vi "Start Sync.vi"(8 "error in (no error)":errorcluster, 10 "current time":timestamp, 11 "gRPC Server in":refnum<class "HVC8.lvclass">) -> (0 "error out":errorcluster, 3 "gRPC Server out":refnum<class "HVC8.lvclass">)   [LabVIEW 2019, in "HVC8.lvlib" / "HVC8.lvclass"]
uses:
  HVC8.lvclass
  DIOSessions.ctl
  DISession.ctl
  DOSession.ctl
  HVC8.lvclass/HVC8.ctl
  RPC Messages/measurementservice_QueryResponse/measurementservice_QueryResponse_Data.ctl
  RPC Messages/measurementservice_DIOpenSessionResponse/measurementservice_DIOpenSessionResponse_Data.ctl
  RPC Messages/measurementservice_ErrorOut/measurementservice_ErrorOut_Data.ctl
  RPC Messages/measurementservice_ReadDIResponse/measurementservice_ReadDIResponse_Data.ctl
  RPC Messages/measurementservice_DICloseSessionResponse/measurementservice_DICloseSessionResponse_Data.ctl
  RPC Messages/measurementservice_DOOpenSessionResponse/measurementservice_DOOpenSessionResponse_Data.ctl
  RPC Messages/measurementservice_DOCloseSessionResponse/measurementservice_DOCloseSessionResponse_Data.ctl
  RPC Messages/measurementservice_WriteDOResponse/measurementservice_WriteDOResponse_Data.ctl
  <vilib>/DAQmx/read.llb/DAQmx Read (Digital 1D Bool 1Chan 1Samp).vi
  <vilib>/DAQmx/write.llb/DAQmx Write (Digital 1D Bool 1Chan 1Samp).vi
  <vilib>/DAQmx/create/channels.llb/DAQmx Create Channel (DI-Digital Input).vi
  <vilib>/DAQmx/miscellaneous.llb/DAQmx Fill In Error Info.vi
  <vilib>/DAQmx/create/channels.llb/DAQmx Create Channel (DO-Digital Output).vi
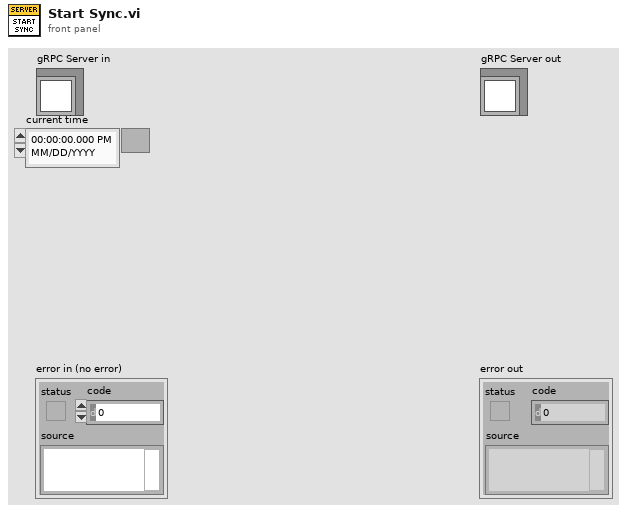
[diagram p1: front panel]
types:
  T1 = typedef "HVC8.lvlib/HVC8.lvclass/DIOSessions.ctl" = cluster{"Array of DI Sessions":T2[], "Array of DO Sessions":T3[]}
  T2 = typedef "HVC8.lvlib/HVC8.lvclass/DISession.ctl" = cluster{"DI Task":refnum<k21>, "DISessionName":string}
  T3 = typedef "HVC8.lvlib/HVC8.lvclass/DOSession.ctl" = cluster{"DOTask":refnum<k21>, "DOSessionName":string}
  T4 = typedef "HVC8.lvlib/HVC8.lvclass/measurementservice_QueryResponse_Data.ctl" = cluster{"message":string, "status":i32}
  T5 = typedef "HVC8.lvlib/HVC8.lvclass/measurementservice_ErrorOut_Data.ctl" = cluster{"errCode":i32, "errMessage":string}
  T6 = typedef "HVC8.lvlib/HVC8.lvclass/measurementservice_DIOpenSessionResponse_Data.ctl" = cluster{"DISessionName":string, "error":T5}
  T7 = typedef "HVC8.lvlib/HVC8.lvclass/measurementservice_ReadDIResponse_Data.ctl" = cluster{"DIOSessionName":string, "DIData":bool[], "error":T5}
  T8 = typedef "HVC8.lvlib/HVC8.lvclass/measurementservice_DICloseSessionResponse_Data.ctl" = cluster{"error":T5}
  T9 = typedef "HVC8.lvlib/HVC8.lvclass/measurementservice_DOOpenSessionResponse_Data.ctl" = cluster{"DOSessionName":string, "error":T5}
  T10 = typedef "HVC8.lvlib/HVC8.lvclass/measurementservice_DOCloseSessionResponse_Data.ctl" = cluster{"error":T5}
  T11 = typedef "HVC8.lvlib/HVC8.lvclass/measurementservice_WriteDOResponse_Data.ctl" = cluster{"DIOSessionName":string, "error":T5}
  T12 = typedef "HVC8.lvlib/HVC8.lvclass/Server gRPC UEs.ctl" = cluster{"Invoke gRPC UE":refnum<user-event>, "Query gRPC UE":refnum<user-event>, "Register gRPC UE":refnum<user-event>, "OpenDISession gRPC UE":refnum<user-event>, "OpenDOSession gRPC UE":refnum<user-event>, "ReadDI gRPC UE":refnum<user-event>, "WriteDO gRPC UE":refnum<user-event>, "CloseDISession gRPC UE":refnum<user-event>, "CloseDOSession gRPC UE":refnum<user-event>}
  T13 = typedef "HVC8.lvlib/gprc-lvsupport.lvlib/grpcId.ctl" = u64
  T14 = typedef "HVC8.lvlib/HVC8.lvclass/measurementservice_QueryRequest_Data.ctl" = cluster{"query":string}
  T15 = typedef "HVC8.lvlib/HVC8.lvclass/measurementservice_DIOpenSessionRequest_Data.ctl" = cluster{"DISessionName":string, "DIlines":string}
  T16 = typedef "HVC8.lvlib/HVC8.lvclass/measurementservice_ReadDIRequest_Data.ctl" = cluster{"DIOSessionName":string}
  T17 = typedef "HVC8.lvlib/HVC8.lvclass/measurementservice_DICloseSessionRequest_Data.ctl" = cluster{"DISessionName":string}
  T18 = typedef "HVC8.lvlib/HVC8.lvclass/measurementservice_DOOpenSessionRequest_Data.ctl" = cluster{"DOSessionName":string, "DOlines":string}
  T19 = typedef "HVC8.lvlib/HVC8.lvclass/measurementservice_DOCloseSessionRequest_Data.ctl" = cluster{"DOSessionName":string}
  T20 = typedef "HVC8.lvlib/HVC8.lvclass/measurementservice_WriteDORequest_Data.ctl" = cluster{"DIOSessionName":string, "DOData":bool[]}
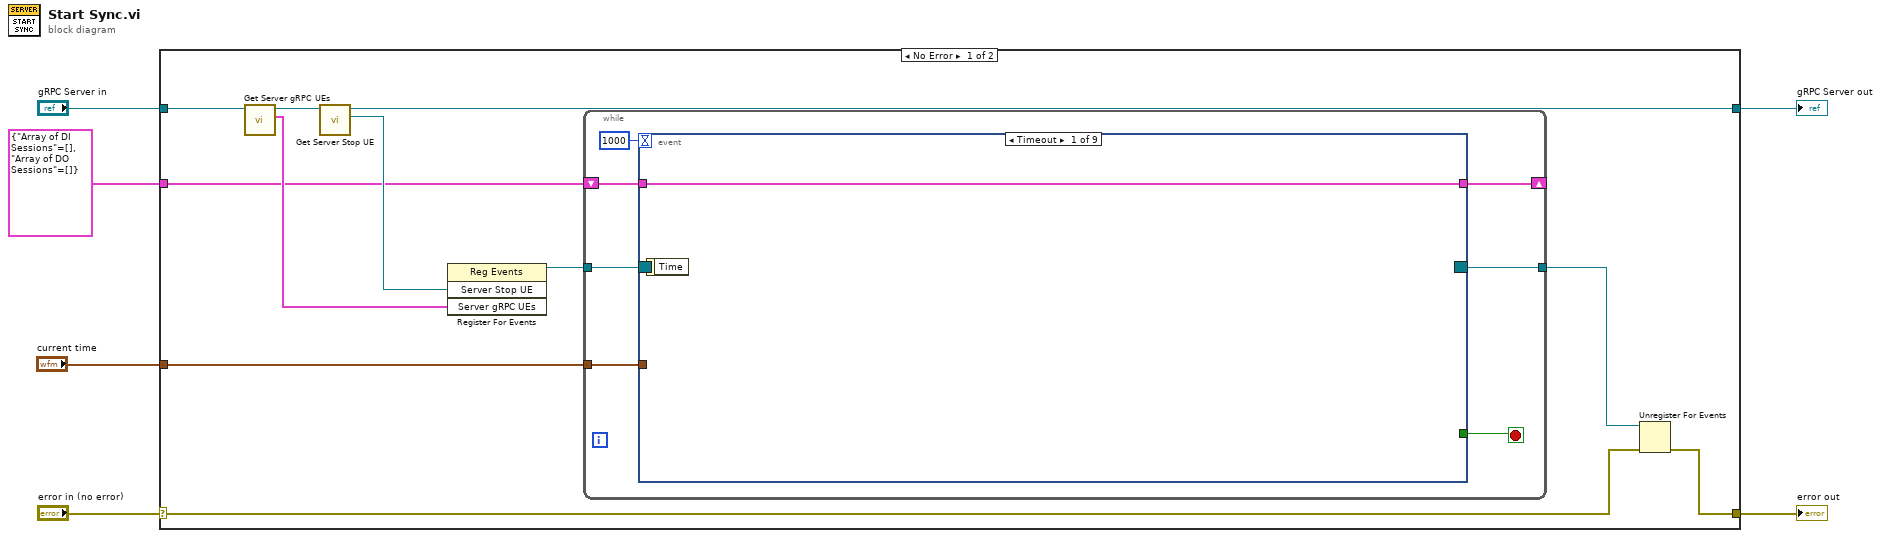
[diagram p0: block diagram]
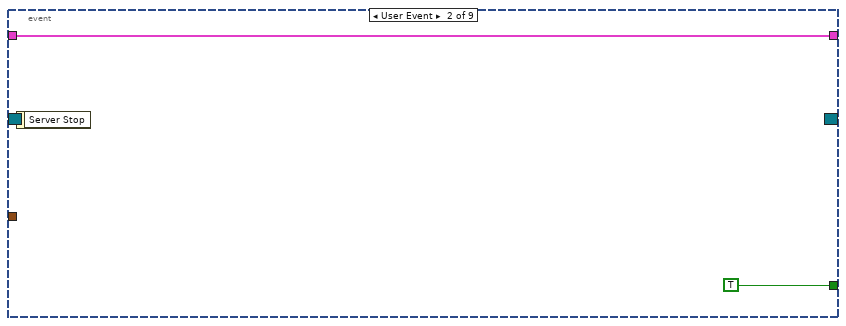
[diagram p2: hidden frame]
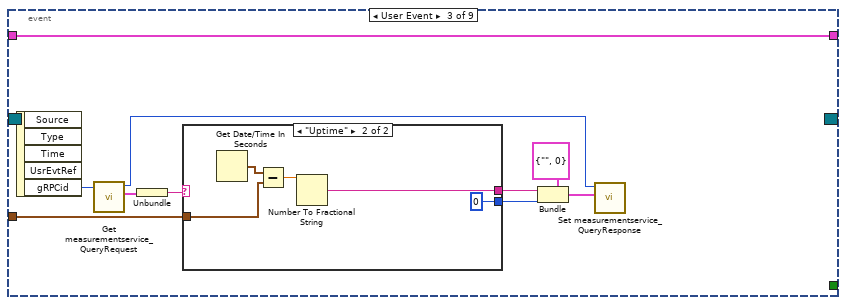
[diagram p3: hidden frame]
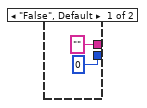
[diagram p4: hidden frame]
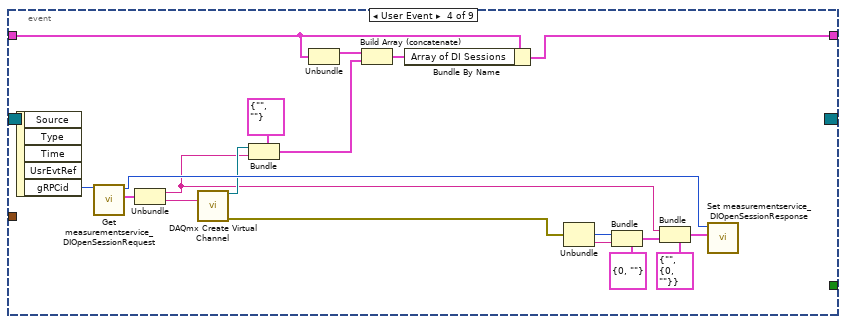
[diagram p5: hidden frame]
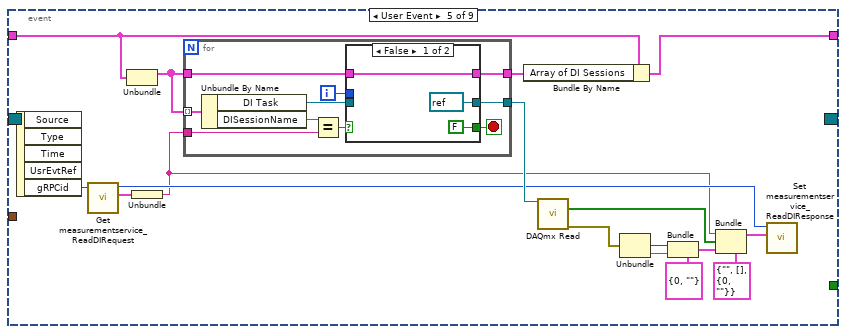
[diagram p6: hidden frame]
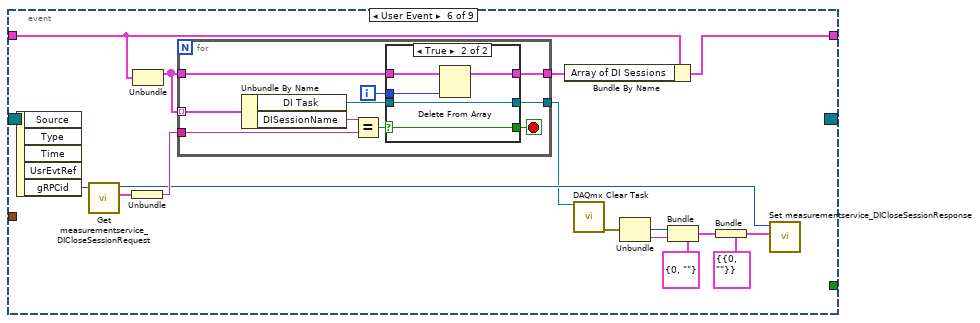
[diagram p8: hidden frame]
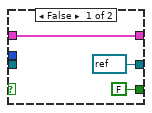
[diagram p9: hidden frame]
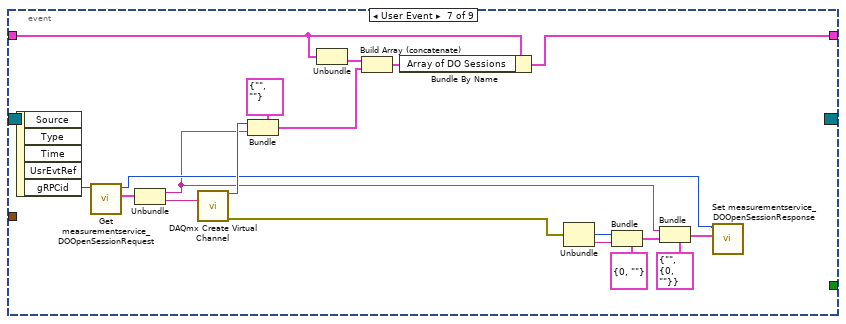
[diagram p10: hidden frame]
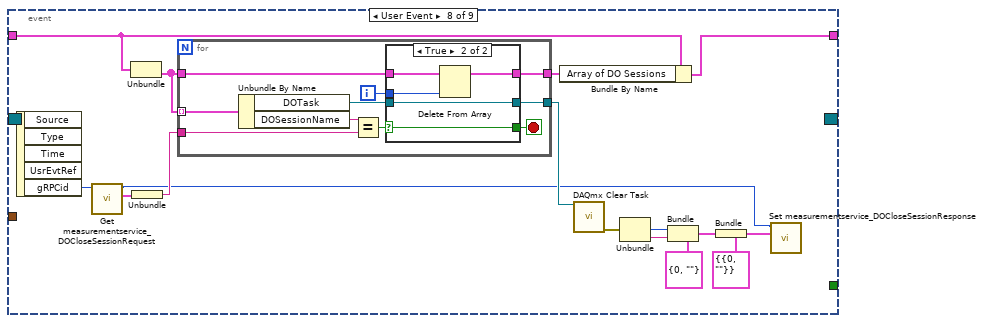
[diagram p11: hidden frame]
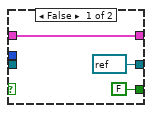
[diagram p12: hidden frame]
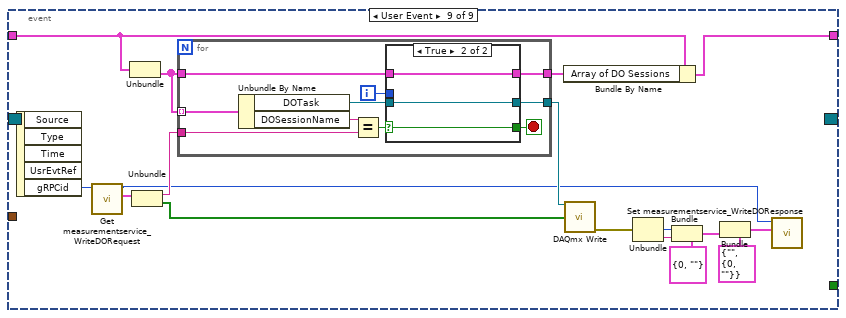
[diagram p13: hidden frame]
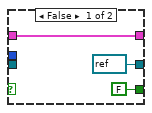
[diagram p14: hidden frame]
diagram:
  n1 = case shown="No Error" "error in (no error)" {
    selector: "error in (no error)" -> [w10 w218]
    tunnel: [w9 w218] -> w5
    tunnel: [w13 w217] -> w3
    tunnel: "gRPC Server in" -> [w17 w217]
    tunnel: "current time" -> [w8 _]
    tunnel: T1 {"Array of DI Sessions"=[], "Array of DO Sessions"=[]} -> [w7 _]
    frame No Error {
      n2 = call "Get Server gRPC UEs.vi"("OOP Server in"=w17) -> ("Server gRPC UEs"=w14:T12, "OOP Server out"=w16:refnum<class "HVC8.lvclass">)  [unwired: 9 in]
      n3 = call "Get Server Stop UE.vi"("OOP Server in"=w16) -> ("Server Stop UE"=w15:refnum<user-event>, "OOP Server out"=w13:refnum<class "HVC8.lvclass">)  [unwired: 9 in]
      n4 = register-events(w15, w14) -> (reference out=w12:refnum<event-registration>)  [unwired: 2 in, 1 out]
      n5 = while {
        tunnel: w12 -> [w24]
        tunnel: [w22] -> w11
        tunnel: w8 -> [w20]
        shift-right: [w18] -> _
        shift-left: w7 -> [w19]
        stop <- w23 stop-if-true
        n6 = event "RPC Methods Event Structure" shown="[0] Timeout" {
          selector: w24 -> [_ _ _ _ _ _ _ _ _]
          dyn-events: [_ _ _ _ _ _ _ _ _] -> w22
          timeout: 1000 -> [_ _ _ _ _ _ _ _ _]
          tunnel: [_ TRUE _ _ _ _ _ _ _] -> w23
          tunnel: w20 -> [_ _ w31 _ _ _ _ _ _]
          tunnel: w19 -> [w25 w26 w28 w47 w66 w99 w131 w152 w185]
          tunnel: [w25 w26 w28 w46 w65 w98 w133 w151 w184] -> w18
          event Timeout {
            n7 = event-data() -> ()  [unwired: 1 in, 1 out]
          }
          event User Event {
            n8 = event-data() -> ()  [unwired: 1 in, 1 out]
          }
          event User Event {
            n9 = event-data() -> ("gRPCid"=w35:T13)  [unwired: 1 in, 4 out]
            n10 = call "Get measurementservice_QueryRequest.vi"("gRPCid"=w35) -> ("Message Data"=w34:T14, "gRPCid out"=w33:T13)  [unwired: 8 in, 1 out]
            n11 = Unbundle(w34) -> ("query"=w32:string)
            n12 = case shown="\"Uptime\"" w32 {
              tunnel: w31 -> [_ w43]
              tunnel: ["" w41] -> w30
              tunnel: [0 ("status") 0 ("status")] -> w29
              frame "False", Default {
              }
              frame "Uptime" {
                n13 = Get Date/Time In Seconds() -> (seconds since 1Jan1904=w44:timestamp)
                n14 = Subtract(x=w44, y=w43) -> (x-y=w42:dbl)
                n15 = Number To Fractional String(number=w42) -> (F-format string=w41:string)  [unwired: 3 in]
              }
            }
            n16 = Bundle(cluster=T4 {"message"="", "status"=0} ("measurementservice_QueryResponse_Data"), "message"=w30, "status"=w29) -> (w36:T4)
            n17 = call "Set measurementservice_QueryResponse.vi"("Message Data"=w36, "gRPCid"=w33) -> ()  [unwired: 9 in, 1 out]
          }
          event User Event {
            n18 = event-data() -> ("gRPCid"=w59:T13)  [unwired: 1 in, 4 out]
            n19 = call "Get measurementservice_DIOpenSessionRequest.vi"("gRPCid"=w59) -> ("Message Data"=w58:T15, "gRPCid out"=w57:T13)  [unwired: 8 in, 1 out]
            n20 = Unbundle(w58) -> ("DISessionName"=w48:string, "DIlines"=w56:string)
            n21 = call-poly <vilib>:"DAQmx Create Virtual Channel.vi"("lines"=w56) -> ("task out"=w49:refnum<k21>, "error out"=w55:errorcluster)  [unwired: 13 in]
            n22 = Bundle(cluster=T2 {"DI Task"="", "DISessionName"=""}, "DI Task"=w49, "DISessionName"=w48) -> (w50:T2)
            n23 = Unbundle(w47) -> ("Array of DI Sessions"=w51:T2[])  [unwired: 1 out]
            n24 = Build Array (concatenate)(w51, w50) -> (w45:T2[])
            n25 = Bundle By Name(cluster=w47, "Array of DI Sessions"=w45) -> (w46:T1)
            n26 = Unbundle(w55) -> ("code"=w54:i32, "source"=w53:string)  [unwired: 1 out]
            n27 = Bundle(cluster=T5 {"errCode"=0, "errMessage"=""} ("error"), "errCode"=w54, "errMessage"=w53) -> (w60:T5)
            n28 = Bundle(cluster=T6 {"DISessionName"="", "error"={"errCode"=0, "errMessage"=""}} ("measurementservice_DIOpenSessionResponse_Data"), "DISessionName"=w48, "error"=w60) -> (w62:T6)
            n29 = call "Set measurementservice_DIOpenSessionResponse.vi"("Message Data"=w62, "gRPCid"=w57) -> ()  [unwired: 9 in, 1 out]
          }
          event User Event {
            n30 = event-data() -> ("gRPCid"=w75:T13)  [unwired: 1 in, 4 out]
            n31 = call "Get measurementservice_ReadDIRequest.vi"("gRPCid"=w75) -> ("Message Data"=w74:T16, "gRPCid out"=w73:T13)  [unwired: 8 in, 1 out]
            n32 = Unbundle(w66) -> ("Array of DI Sessions"=w78:T2[])  [unwired: 1 out]
            n33 = Unbundle(w74) -> ("DIOSessionName"=w67:string)
            n34 = for {
              tunnel: w78 -> [w85] mode=indexing
              tunnel: w67 -> [w90]
              tunnel: [w86] -> w77
              tunnel: w78 -> [w84]
              tunnel: [w83] -> w64
              i -> [w81]
              stop <- w88 stop-if-true
              n35 = Unbundle By Name(w85) -> ("DI Task"=w87:refnum<k21>, "DISessionName"=w82:string)
              n36 = Equal?(x=w82, y=w90) -> (x = y?=w89:bool)
              n37 = case shown="False" w89 {
                selector: w89 -> [_ w96]
                tunnel: [FALSE w96] -> w88
                tunnel: w87 -> [_ w94]
                tunnel: [refnum<k21> refnum ("DI Task") w94] -> w86
                tunnel: w84 -> [w91 w95]
                tunnel: [w91 w95] -> w83
                tunnel: w81 -> [_ _]
                frame False {
                }
                frame True {
                }
              }
            }
            n38 = Bundle By Name(cluster=w66, "Array of DI Sessions"=w64) -> (w65:T1)
            n39 = call-poly <vilib>:"DAQmx Read.vi"("task/channels in"=w77) -> ("data"=w68:bool[], "error out"=w76:errorcluster)  [unwired: 12 in, 1 out]
            n40 = Unbundle(w76) -> ("code"=w80:i32, "source"=w79:string)  [unwired: 1 out]
            n41 = Bundle(cluster=T5 {"errCode"=0, "errMessage"=""} ("error"), "errCode"=w80, "errMessage"=w79) -> (w69:T5)
            n42 = Bundle(cluster=T7 {"DIOSessionName"="", "DIData"=[], "error"={"errCode"=0, "errMessage"=""}} ("measurementservice_ReadDIResponse_Data"), "DIOSessionName"=w67, "DIData"=w68, "error"=w69) -> (w72:T7)
            n43 = call "Set measurementservice_ReadDIResponse.vi"("Message Data"=w72, "gRPCid"=w73) -> ()  [unwired: 9 in, 1 out]
          }
          event User Event {
            n44 = event-data() -> ("gRPCid"=w109:T13)  [unwired: 1 in, 4 out]
            n45 = call "Get measurementservice_DICloseSessionRequest.vi"("gRPCid"=w109) -> ("Message Data"=w108:T17, "gRPCid out"=w106:T13)  [unwired: 8 in, 1 out]
            n46 = Unbundle(w108) -> ("DISessionName"=w107:string)
            n47 = Unbundle(w99) -> ("Array of DI Sessions"=w100:T2[])  [unwired: 1 out]
            n48 = for {
              tunnel: w100 -> [w117] mode=indexing
              tunnel: w107 -> [w122]
              tunnel: [w118] -> w101
              tunnel: w100 -> [w116]
              tunnel: [w115] -> w97
              i -> [w113]
              stop <- w120 stop-if-true
              n49 = Unbundle By Name(w117) -> ("DI Task"=w119:refnum<k21>, "DISessionName"=w114:string)
              n50 = Equal?(x=w114, y=w122) -> (x = y?=w121:bool)
              n51 = case shown="True" w121 {
                selector: w121 -> [_ w130]
                tunnel: [FALSE w130] -> w120
                tunnel: w119 -> [_ w128]
                tunnel: [refnum<k21> refnum ("DI Task") w128] -> w118
                tunnel: w116 -> [w123 w129]
                tunnel: [w123 w126] -> w115
                tunnel: w113 -> [_ w127]
                frame False {
                }
                frame True {
                  n52 = Delete From Array(array=w129, index=w127) -> (array with subset deleted=w126:T2[])  [unwired: 1 in, 1 out]
                }
              }
            }
            n53 = Bundle By Name(cluster=w99, "Array of DI Sessions"=w97) -> (w98:T1)
            n54 = call <vilib>:"DAQmx Clear Task.vi"("task in"=w101) -> ("error out"=w110:errorcluster)  [unwired: 14 in]
            n55 = Unbundle(w110) -> ("code"=w112:i32, "source"=w111:string)  [unwired: 1 out]
            n56 = Bundle(cluster=T5 {"errCode"=0, "errMessage"=""} ("error"), "errCode"=w112, "errMessage"=w111) -> (w102:T5)
            n57 = Bundle(cluster=T8 {"error"={"errCode"=0, "errMessage"=""}} ("measurementservice_DICloseSessionResponse_Data"), "error"=w102) -> (w105:T8)
            n58 = call "Set measurementservice_DICloseSessionResponse.vi"("Message Data"=w105, "gRPCid"=w106) -> ()  [unwired: 9 in, 1 out]
          }
          event User Event {
            n59 = event-data() -> ("gRPCid"=w144:T13)  [unwired: 1 in, 4 out]
            n60 = call "Get measurementservice_DOOpenSessionRequest.vi"("gRPCid"=w144) -> ("Message Data"=w143:T18, "gRPCid out"=w139:T13)  [unwired: 8 in, 1 out]
            n61 = Unbundle(w143) -> ("DOSessionName"=w134:string, "DOlines"=w149:string)
            n62 = call-poly <vilib>:"DAQmx Create Virtual Channel.vi"("lines"=w149) -> ("task out"=w145:refnum<k21>, "error out"=w148:errorcluster)  [unwired: 13 in]
            n63 = Bundle(cluster=T3 {"DOTask"="", "DOSessionName"=""} ("output cluster"), "DOTask"=w145, "DOSessionName"=w134) -> (w140:T3)
            n64 = Unbundle(w131) -> ("Array of DO Sessions"=w142:T3[])  [unwired: 1 out]
            n65 = Build Array (concatenate)(w142, w140) -> (w132:T3[])
            n66 = Bundle By Name(cluster=w131, "Array of DO Sessions"=w132) -> (w133:T1)
            n67 = Unbundle(w148) -> ("code"=w147:i32, "source"=w146:string)  [unwired: 1 out]
            n68 = Bundle(cluster=T5 {"errCode"=0, "errMessage"=""} ("error"), "errCode"=w147, "errMessage"=w146) -> (w135:T5)
            n69 = Bundle(cluster=T9 {"DOSessionName"="", "error"={"errCode"=0, "errMessage"=""}} ("measurementservice_DOOpenSessionResponse_Data"), "DOSessionName"=w134, "error"=w135) -> (w138:T9)
            n70 = call "Set measurementservice_DOOpenSessionResponse.vi"("Message Data"=w138, "gRPCid"=w139) -> ()  [unwired: 9 in, 1 out]
          }
          event User Event {
            n71 = event-data() -> ("gRPCid"=w160:T13)  [unwired: 1 in, 4 out]
            n72 = call "Get measurementservice_DOCloseSessionRequest.vi"("gRPCid"=w160) -> ("Message Data"=w159:T19, "gRPCid out"=w158:T13)  [unwired: 8 in, 1 out]
            n73 = Unbundle(w152) -> ("Array of DO Sessions"=w153:T3[])  [unwired: 1 out]
            n74 = Unbundle(w159) -> ("DOSessionName"=w162:string)
            n75 = for {
              tunnel: w153 -> [w170] mode=indexing
              tunnel: w162 -> [w175]
              tunnel: [w171] -> w161
              tunnel: w153 -> [w169]
              tunnel: [w168] -> w150
              i -> [w166]
              stop <- w173 stop-if-true
              n76 = Unbundle By Name(w170) -> ("DOTask"=w172:refnum<k21>, "DOSessionName"=w167:string)
              n77 = Equal?(x=w167, y=w175) -> (x = y?=w174:bool)
              n78 = case shown="True" w174 {
                selector: w174 -> [_ w183]
                tunnel: [FALSE w183] -> w173
                tunnel: w172 -> [_ w181]
                tunnel: [refnum<k21> refnum ("DI Task") w181] -> w171
                tunnel: w169 -> [w176 w182]
                tunnel: [w176 w179] -> w168
                tunnel: w166 -> [_ w180]
                frame False {
                }
                frame True {
                  n79 = Delete From Array(array=w182, index=w180) -> (array with subset deleted=w179:T3[])  [unwired: 1 in, 1 out]
                }
              }
            }
            n80 = Bundle By Name(cluster=w152, "Array of DO Sessions"=w150) -> (w151:T1)
            n81 = call <vilib>:"DAQmx Clear Task.vi"("task in"=w161) -> ("error out"=w163:errorcluster)  [unwired: 14 in]
            n82 = Unbundle(w163) -> ("code"=w165:i32, "source"=w164:string)  [unwired: 1 out]
            n83 = Bundle(cluster=T5 {"errCode"=0, "errMessage"=""} ("error"), "errCode"=w165, "errMessage"=w164) -> (w154:T5)
            n84 = Bundle(cluster=T10 {"error"={"errCode"=0, "errMessage"=""}} ("measurementservice_DOCloseSessionResponse_Data"), "error"=w154) -> (w156:T10)
            n85 = call "Set measurementservice_DOCloseSessionResponse.vi"("Message Data"=w156, "gRPCid"=w158) -> ()  [unwired: 9 in, 1 out]
          }
          event User Event {
            n86 = event-data() -> ("gRPCid"=w196:T13)  [unwired: 1 in, 4 out]
            n87 = call "Get measurementservice_WriteDORequest.vi"("gRPCid"=w196) -> ("Message Data"=w195:T20, "gRPCid out"=w191:T13)  [unwired: 8 in, 1 out]
            n88 = Unbundle(w185) -> ("Array of DO Sessions"=w197:T3[])  [unwired: 1 out]
            n89 = Unbundle(w195) -> ("DIOSessionName"=w198:string, "DOData"=w192:bool[])
            n90 = for {
              tunnel: w197 -> [w205] mode=indexing
              tunnel: w198 -> [w210]
              tunnel: [w206] -> w193
              tunnel: w197 -> [w204]
              tunnel: [w203] -> w186
              i -> [w201]
              stop <- w208 stop-if-true
              n91 = Unbundle By Name(w205) -> ("DOTask"=w207:refnum<k21>, "DOSessionName"=w202:string)
              n92 = Equal?(x=w202, y=w210) -> (x = y?=w209:bool)
              n93 = case shown="True" w209 {
                selector: w209 -> [_ w216]
                tunnel: [FALSE w216] -> w208
                tunnel: w207 -> [_ w214]
                tunnel: [refnum<k21> refnum ("DI Task") w214] -> w206
                tunnel: w204 -> [w211 w215]
                tunnel: [w211 w215] -> w203
                tunnel: w201 -> [_ _]
                frame False {
                }
                frame True {
                }
              }
            }
            n94 = Bundle By Name(cluster=w185, "Array of DO Sessions"=w186) -> (w184:T1)
            n95 = call-poly <vilib>:"DAQmx Write.vi"("task/channels in"=w193, "data"=w192) -> ("error out"=w194:errorcluster)  [unwired: 11 in, 2 out]
            n96 = Unbundle(w194) -> ("code"=w200:i32, "source"=w199:string)  [unwired: 1 out]
            n97 = Bundle(cluster=T5 {"errCode"=0, "errMessage"=""} ("error"), "errCode"=w200, "errMessage"=w199) -> (w187:T5)
            n98 = Bundle(cluster=T11 {"DIOSessionName"="", "error"={"errCode"=0, "errMessage"=""}} ("measurementservice_WriteDOResponse_Data"), "error"=w187) -> (w190:T11)  [unwired: 1 in]
            n99 = call "Set measurementservice_WriteDOResponse.vi"("Message Data"=w190, "gRPCid"=w191) -> ()  [unwired: 9 in, 1 out]
          }
        }
      }
      n100 = Unregister For Events(event registration refnum=w11, error in=w10) -> (error out=w9:errorcluster)
    }
    frame Error {
    }
  }
  "error out" <- w5
  "gRPC Server out" <- w3
